vi "orginlab-keitley.vi"(6 "\\I-V-2.opj":string, 7 "Zaman":dbl[](array[numeric]), 9 "[Book1]Sheet1":string, 10 "Akým":dbl[](array[numeric]), 11 "Gerilim":dbl[](array[numeric])) -> ()   [LabVIEW 2020]
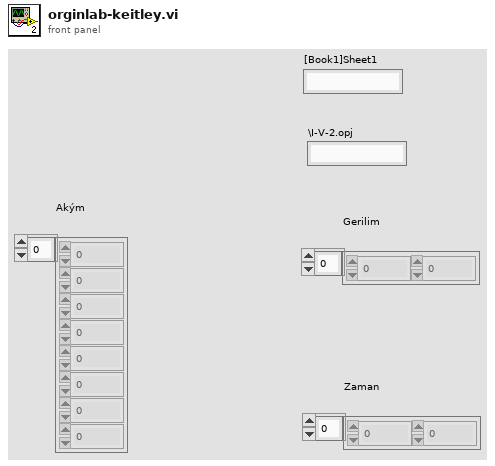
[diagram p1: front panel]
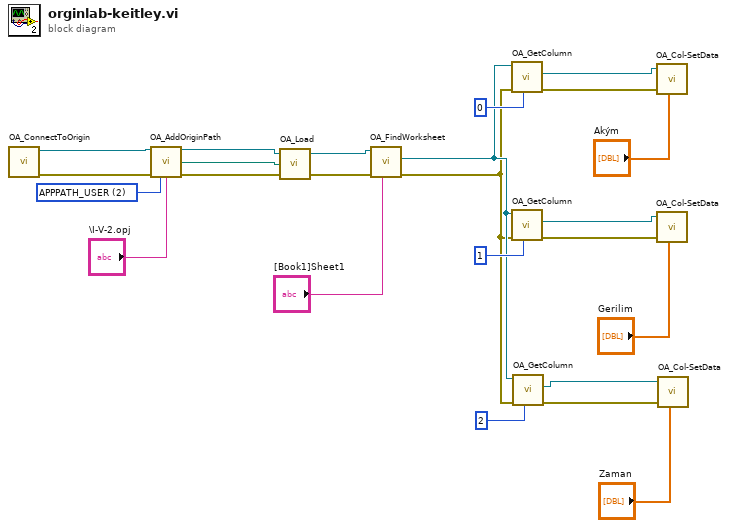
[diagram p0: block diagram]
diagram:
  w12 = 2 items=["APPPATH_USER"=2, "APPPATH_GROUP"=3, "APPPATH_PROGRAM"=4] ("Type")
  n1 = call "OA_ConnectToOrigin.vi"() -> ("error out"=w13:errorcluster, "Origin.IOApplication"=w14:refnum<k7>)  [unwired: 8 in]
  n2 = call "OA_AddOriginPath.vi"("Origin.IOApplication"=w14, "error in (no error)"=w13, "Type"=w12, "Filename"="\\I-V-2.opj") -> ("Origin.IOApplication"=w10:refnum<k7>, "path out"=w8:path, "error out"=w9:errorcluster)  [unwired: 9 in]
  n3 = call "OA_Load.vi"("error in (no error)"=w9, "Path"=w8, "Origin.IOApplication"=w10) -> ("error out"=w17:errorcluster, "Origin.IOApplication"=w16:refnum<k7>)  [unwired: 1 out]
  n4 = call "OA_FindWorksheet.vi"("Name"="[Book1]Sheet1", "error in (no error)"=w17, "Origin.IOApplication"=w16) -> ("error out"=w2:errorcluster, "Origin.Worksheet"=w3:refnum<k7>)  [unwired: 6 in, 1 out]
  n5 = call "OA_GetColumn.vi"("Column Name/Index"=0, "error in (no error)"=w2, "Origin.Worksheet"=w3) -> ("error out"=w20:errorcluster, "Origin.Column"=w19:refnum<k7>)  [unwired: 6 in, 1 out]
  n6 = call "OA_GetColumn.vi"("Column Name/Index"=1, "error in (no error)"=w2, "Origin.Worksheet"=w3) -> ("error out"=w22:errorcluster, "Origin.Column"=w23:refnum<k7>)  [unwired: 6 in, 1 out]
  n7 = call "OA_GetColumn.vi"("Column Name/Index"=2, "error in (no error)"=w2, "Origin.Worksheet"=w3) -> ("error out"=w5:errorcluster, "Origin.Column"=w1:refnum<k7>)  [unwired: 6 in, 1 out]
  n8 = call "OA_Col-SetData.vi"("Origin.Column"=w19, "error in (no error)"=w20, "data"="Akým") -> ()  [unwired: 4 in, 3 out]
  n9 = call "OA_Col-SetData.vi"("Origin.Column"=w23, "error in (no error)"=w22, "data"="Gerilim") -> ()  [unwired: 4 in, 3 out]
  n10 = call "OA_Col-SetData.vi"("Origin.Column"=w1, "error in (no error)"=w5, "data"="Zaman") -> ()  [unwired: 4 in, 3 out]
